vi "CC Parse Declination.vi"(8 "error in (no error)":errorcluster, 11 "Declination string":string) -> (0 "error out":errorcluster, 2 "Angle":dbl, 3 "Declination":T1)   [LabVIEW 2021]
uses:
  <vilib>/regexp/Match Regular Expression.xnode
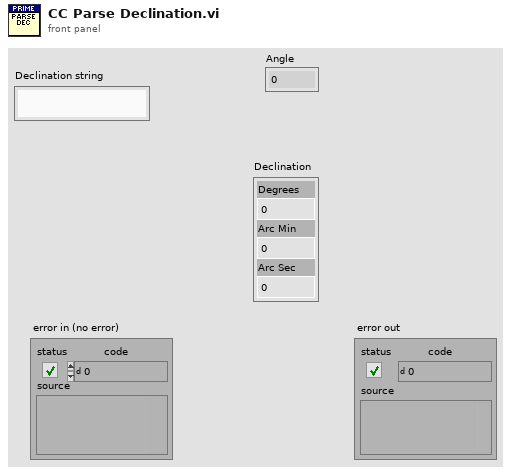
[diagram p1: front panel]
types:
  T1 = cluster{"Degrees":dbl, "Arc Min":dbl, "Arc Sec":dbl}
  T2 = cluster{"hours":dbl, "Minutes":dbl, "seconds":dbl}
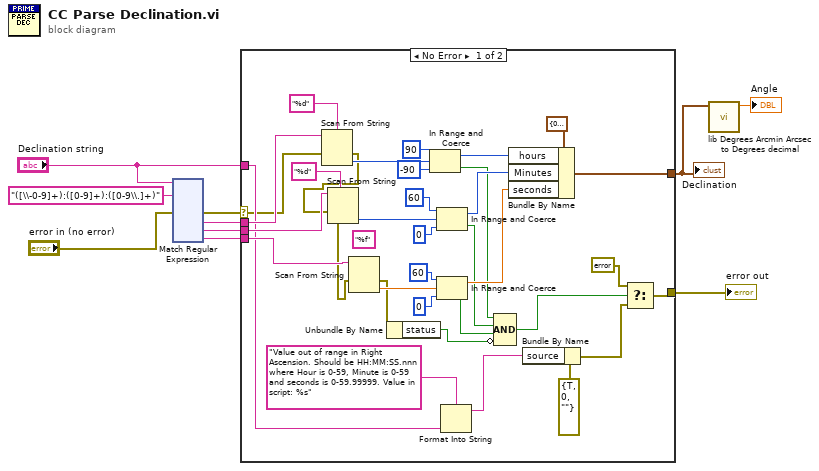
[diagram p0: block diagram]
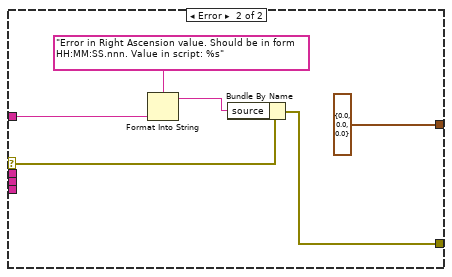
[diagram p2: hidden frame]
diagram:
  n1 = xnode "Match Regular Expression"("input string"="Declination string", "regular expression"="([\\-0-9]+):([0-9]+):([0-9\\.]+)", "error in"="error in (no error)") -> ("error out"=w5:errorcluster, "submatch 1"=w9:string, "submatch 2"=w8:string, "submatch 3"=w7:string)  [unwired: 3 in, 4 out]
  n2 = case shown="No Error" w5 {
    selector: w5 -> [w15 w49]
    tunnel: w9 -> [w45 _]
    tunnel: w8 -> [w42 _]
    tunnel: w7 -> [w41 _]
    tunnel: [w27 T2 {"hours"=0.0, "Minutes"=0.0, "seconds"=0.0} ("Right Ascension 2")] -> w2
    tunnel: "Declination string" -> [w18 w50]
    tunnel: [w16 w47] -> w3
    frame No Error {
      (unwired) "%f" ("format string")
      n3 = Scan From String(format string="%d", input string=w45, error in=w15) -> (error out=w14:errorcluster, output 1=w40:i32)  [unwired: 2 in, 2 out]
      n4 = Scan From String(format string="%d", input string=w42, error in=w14) -> (error out=w13:errorcluster, output 1=w37:i32)  [unwired: 2 in, 2 out]
      n5 = Scan From String(input string=w41, error in=w13) -> (error out=w12:errorcluster, output 1=w32:dbl)  [unwired: 3 in, 2 out]
      n6 = Unbundle By Name(w12) -> ("status"=w11:bool)
      n7 = In Range and Coerce(upper limit=90, x=w40, lower limit=-90) -> (coerced(x)=w30:i32, In Range?=w26:bool)
      n8 = In Range and Coerce(upper limit=60, x=w37, lower limit=0) -> (coerced(x)=w29:i32, In Range?=w25:bool)
      n9 = In Range and Coerce(upper limit=60, x=w32, lower limit=0) -> (coerced(x)=w28:dbl, In Range?=w24:bool)
      n10 = Format Into String(format string="Value out of range in Right Ascension. Should be HH:MM:SS.nnn where Hour is 0-59, Minute is 0-59 and seconds is 0-59.99999. Value in script: %s", w18) -> (resulting string=w17:string)  [unwired: 2 in, 1 out]
      n11 = Compound Arithmetic op=AND(w26, w25, w24, invert w11) -> (w23:bool)
      n12 = Bundle By Name(cluster=T2 {"hours"=0.0, "Minutes"=0.0, "seconds"=0.0} ("Right Ascension 2"), "hours"=w30, "Minutes"=w29, "seconds"=w28) -> (w27:T2)
      n13 = Bundle By Name(cluster=errorcluster {"status"=TRUE, "code"=0, "source"=""} ("error out"), "source"=w17) -> (w21:errorcluster)
      n14 = Select(t=errorcluster {"status"=FALSE, "code"=0, "source"=""}, s=w23, f=w21) -> (s? t:f=w16:errorcluster)
    }
    frame Error {
      n15 = Format Into String(format string="Error in Right Ascension value. Should be in form HH:MM:SS.nnn. Value in script: %s", w50) -> (resulting string=w48:string)  [unwired: 2 in, 1 out]
      n16 = Bundle By Name(cluster=w49, "source"=w48) -> (w47:errorcluster)
    }
  }
  "error out" <- w3
  "Declination" <- w2
  n17 = call "lib Degrees Arcmin Arcsec to Degrees decimal.vi"("Declination"=w2) -> ("Angle"=→"Angle":dbl)  [unwired: 9 in, 1 out]
